vi "Parse Text-Comment-Text.vi"(8 "Error In":errorcluster) -> (0 "Error Out":errorcluster)   [LabVIEW 2018, in "Tests.lvlib" / "Parser.lvlib"]
uses:
  Parser.lvlib
  src/Toolkit/Public/Tokens/Text/Text.lvclass
  src/Toolkit/Public/Readers/String/String.lvclass
  D:/Users/cfield/Code/Field R&D Services/Mustache/trunk/src/Mustache/Public/Readers/Public/Abstract/Abstract.lvclass
  <vilib>/Utility/LVClass/Get LV Class Name.vi
  src/Toolkit/Public/Tokens/Text/API/Read Content.vi
  <vilib>/addons/_JKI Toolkits/Caraya/classes/Assert/Assert Equal_Variant.vi
  <vilib>/addons/_JKI Toolkits/Caraya/classes/Test/Test.lvclass
  src/Toolkit/Public/Parser/Parser.lvclass
  <vilib>/addons/_JKI Toolkits/Caraya/classes/Assert/Assert.lvclass
  Tests.lvlib
  src/Toolkit/Public/Tokens/Abstract/Abstract.lvclass
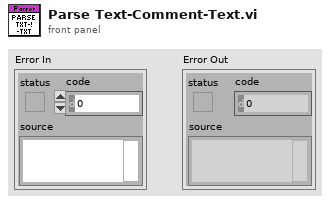
[diagram p1: front panel]
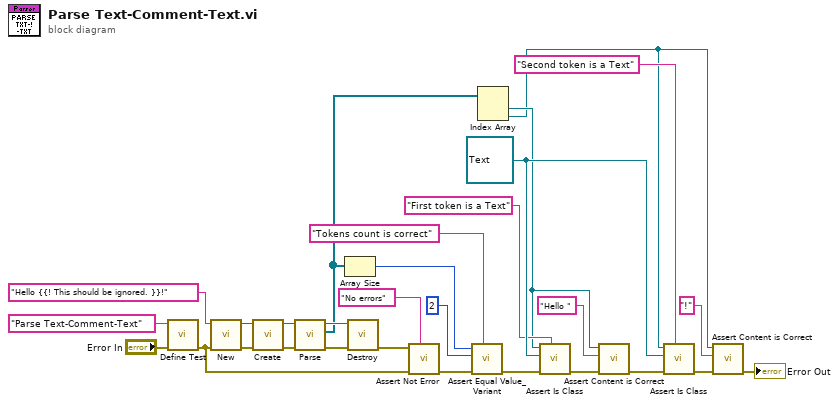
[diagram p0: block diagram]
diagram:
  w8 = refnum<class "Text.lvclass"> refnum ("Mustache.lvlib:Tokens.lvlib:Text.lvclass")
  n1 = call <vilib>:"Define Test.vi"("error in (no error)"="Error In", "Label (VI Title)"="Parse Text-Comment-Text") -> ("error out"=w13:errorcluster)  [unwired: 9 in]
  n2 = call "New.vi"("Error In"=w13, "String"="Hello {{! This should be ignored. }}!" ("format string")) -> ("Error Out"=w26:errorcluster, "String"=w27:refnum<class "String.lvclass">)  [unwired: 8 in]
  n3 = call "Create.vi"("Error In"=w26, "Reader"=w27) -> ("Error Out"=w25:errorcluster, "Parser"=w24:refnum<class "Parser.lvclass">)  [unwired: 8 in]
  n4 = call "Parse.vi"("Error In"=w25, "Parser In"=w24) -> ("Error Out"=w22:errorcluster, "Tokens"=w14:refnum<class "Abstract.lvclass">[], "Parser Out"=w23:refnum<class "Parser.lvclass">)  [unwired: 7 in]
  n5 = Array Size(array=w14) -> (size(s)=w17:i32)
  n6 = call "Destroy.vi"("Error In"=w22, "Parser"=w23) -> ("Error Out"=w21:errorcluster)  [unwired: 9 in]
  n7 = call <vilib>:"Assert Not Error.vi"("Label"="No errors", "error in (no error)"=w13, "Not Error?"=w21) -> ("error out"=w19:errorcluster)  [unwired: 8 in]
  n8 = call <vilib>:"Assert Equal Value_Variant.vi"("Label"="Tokens count is correct", "error in (no error)"=w19, "Y"=2 ("size(s)"), "X"=w17) -> ("error out"=w15:errorcluster)  [unwired: 7 in]
  n9 = Index Array(array=w14) -> (element #1=w3:refnum<class "Abstract.lvclass">, element #2=w2:refnum<class "Abstract.lvclass">)  [unwired: 2 in]
  n10 = call "Assert Is Class.vi"("Label"="First token is a Text", "Error In"=w15, "Expected"=w8, "Actual"=w3) -> ("Error Out"=w12:errorcluster)  [unwired: 7 in]
  n11 = call "Assert Content is Correct.vi"("Error In"=w12, "Expected"="Hello ", "Token"=w3) -> ("Error Out"=w11:errorcluster)  [unwired: 8 in]
  n12 = call "Assert Is Class.vi"("Label"="Second token is a Text", "Error In"=w11, "Expected"=w8, "Actual"=w2) -> ("Error Out"=w10:errorcluster)  [unwired: 7 in]
  n13 = call "Assert Content is Correct.vi"("Error In"=w10, "Expected"="!", "Token"=w2) -> ("Error Out"=→"Error Out":errorcluster)  [unwired: 8 in]
